vi "Create Debug Log.vi"(8 "error in (no error)":errorcluster, 11 "Pre-Push data":u16[](array[numeric])) -> (0 "error out":errorcluster)   [LabVIEW 2016, in "BCI-1553 API.lvlib" / "1553 Component.lvclass"]
uses:
  1553 Component.lvclass
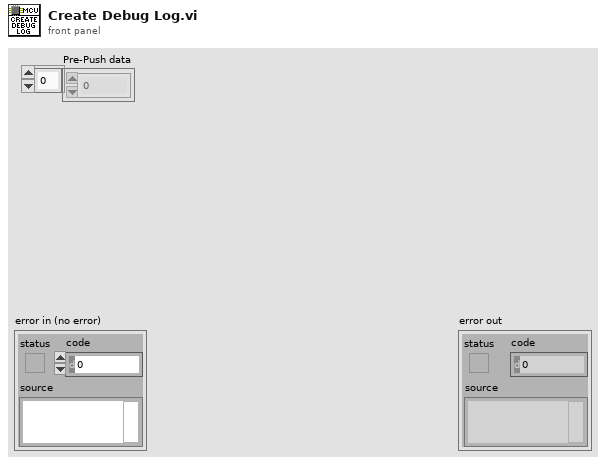
[diagram p1: front panel]
types:
  T1 = enum16{"open", "replace", "create", "open or create", "replace or create", "replace or create with confirmation"}
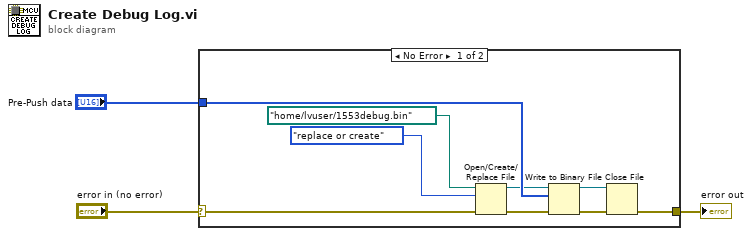
[diagram p0: block diagram]
diagram:
  n1 = case shown="No Error" "error in (no error)" {
    selector: "error in (no error)" -> [w5 w13]
    tunnel: [w9 w13] -> w2
    tunnel: "Pre-Push data" -> [w12 _]
    frame No Error {
      n2 = Open/Create/Replace File(file path (use dialog)=path "/home/lvuser/1553debug.bin", error in=w5, operation (0:open)=T1."replace or create") -> (refnum out=w8:refnum<file>, error out=w4:errorcluster)  [unwired: 3 in, 1 out]
      n3 = Write to Binary File(file (use dialog)=w8, data=w12, error in=w4) -> (refnum out=w11:refnum<file>, error out=w10:errorcluster)  [unwired: 3 in, 1 out]
      n4 = Close File(refnum=w11, error in=w10) -> (error out=w9:errorcluster)  [unwired: 1 out]
    }
    frame Error {
    }
  }
  "error out" <- w2
